vi "RectTBtoRect.vi"(11 "RectTB":T1) -> (3 "rect":T2 caption="矩形")   [LabVIEW 2012, in "Picture Box Tools.lvlib"]
uses:
  Picture Box Tools.lvlib
  RectTB/RectTB.ctl
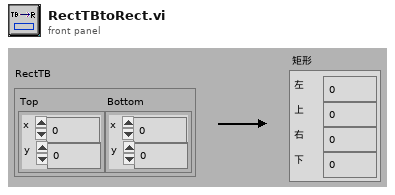
[diagram p1: front panel]
types:
  T1 = typedef "Picture Box Tools.lvlib/RectTB.ctl" = cluster{"Top":cluster{"x":i16, "y":i16}, "Bottom":cluster{"x":i16, "y":i16}}
  T2 = cluster{"left":i16, "top":i16, "right":i16, "bottom":i16}
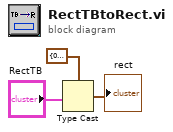
[diagram p0: block diagram]
diagram:
  n1 = Type Cast(type=T2 {"left"=0, "top"=0, "right"=0, "bottom"=0} ("rect"), x="RectTB") -> (*(type *) &x=→"rect":T2)
